vi "IndexName.vi"(8 "ErrorIn(No Error)":errorcluster caption="entrée d'erreur (pas d'erreur)", 10 "ClassArray":string[][](array[string])=[["EG_G5210", "EG_G5210"], ["EG_G5210_1", "EG_G5210"]], 11 "ClassName":string="EG_G5210") -> (0 "sortie d'erreur":errorcluster, 1 "AllInstrNamesArr":string[](array[string]), 2 "ClsInstrNamesArr":string[](array[string]), 3 "Instrument name":string)   [LabVIEW 2019]
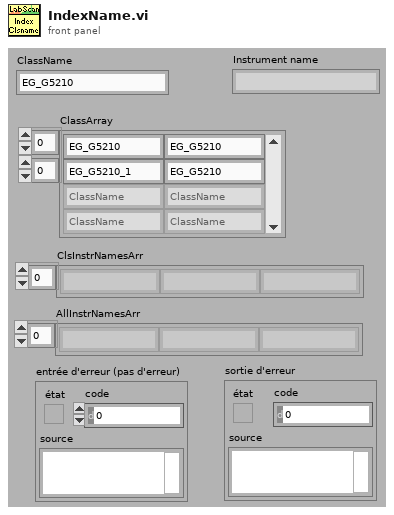
[diagram p1: front panel]
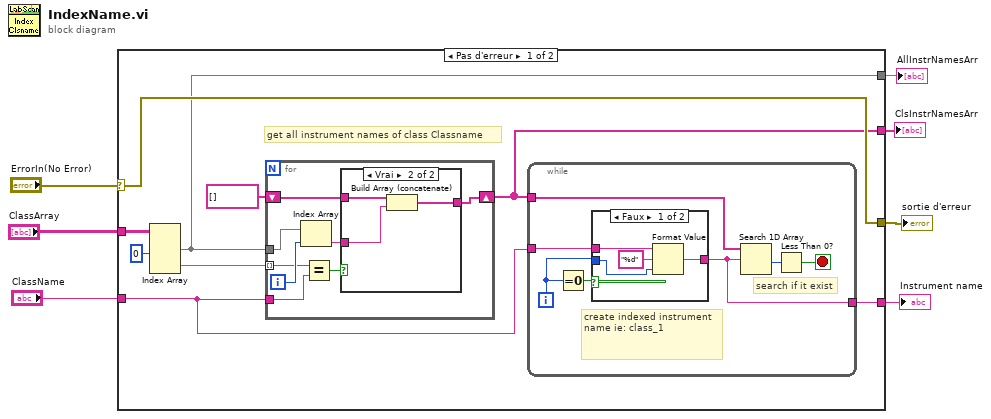
[diagram p0: block diagram]
diagram:
  n1 = case shown="Pas d'erreur" "ErrorIn(No Error)" {
    selector: "ErrorIn(No Error)" -> [w10 w41]
    tunnel: "ClassArray" -> [w15 _]
    tunnel: "ClassName" -> [w12 _]
    tunnel: [w11 _] -> w5
    tunnel: [w10 w41] -> w3
    tunnel: [w9 _] -> w2
    tunnel: [w8 _] -> w1
    frame No Error {
      # "get all instrument names of class Classname"
      n2 = Index Array(array=w15, index (col) #1=0 ("indice désactivé (col)")) -> (element #1=w8:string[], element #2=w14:string[])  [unwired: 3 in]
      n3 = for {
        tunnel: w14 -> [w30] mode=indexing
        tunnel: w8 -> [w34]
        shift-right: [w31] -> w9
        shift-left: string[] [] -> [w35]
        tunnel: w12 -> [w29]
        i -> [w32]
        n4 = Index Array(array=w34, index=w32) -> (element=w33:string)
        n5 = Equal?(x=w30, y=w29) -> (x = y?=w36:bool)
        n6 = case shown="Vrai" w36 {
          tunnel: w35 -> [w37 w40]
          tunnel: w33 -> [_ w39]
          tunnel: [w37 w38] -> w31
          frame False {
          }
          frame True {
            n7 = Build Array (concatenate)(w40, w39) -> (w38:string[])
          }
        }
      }
      n8 = while {
        tunnel: w9 -> [w20]
        tunnel: w12 -> [w22]
        tunnel: [w17] -> w11
        i -> [w21]
        stop <- w18 stop-if-true
        # "search if it exist"
        # "create indexed instrument name ie: class_1"
        n9 = Equal To 0?(x=w21) -> (x = 0?=w23:bool)
        n10 = case shown="Faux" w23 {
          tunnel: w22 -> [w27 w28]
          tunnel: [w24 w28] -> w17
          tunnel: w21 -> [w25 _]
          frame False {
            n11 = Format Value(string ("")=w27, format string="%d" ("chaîne de format"), value (0)=w25) -> (output string=w24:string)
          }
          frame True {
          }
        }
        n12 = Search 1D Array(1D array=w20, element=w17) -> (index of element=w19:i32)  [unwired: 1 in]
        n13 = Less Than 0?(x=w19) -> (x < 0?=w18:bool)
      }
    }
    frame Error {
    }
  }
  "Instrument name" <- w5
  "sortie d'erreur" <- w3
  "ClsInstrNamesArr" <- w2
  "AllInstrNamesArr" <- w1
